vi "Week_4_4.1_Ex-4.vi"() -> ()   [LabVIEW 2015]
panel:
  in  "Gauge":dbl(knob) scale=-360.0..360.0
  out "Active Power":dbl format="%#_13g"
  out "Reactive Power":dbl format="%#_13g"
  out "V RMS":dbl format="%#_13g"
  out "Apparent Power":dbl format="%#_13g"
  out "I-RMS":dbl format="%#_13g"
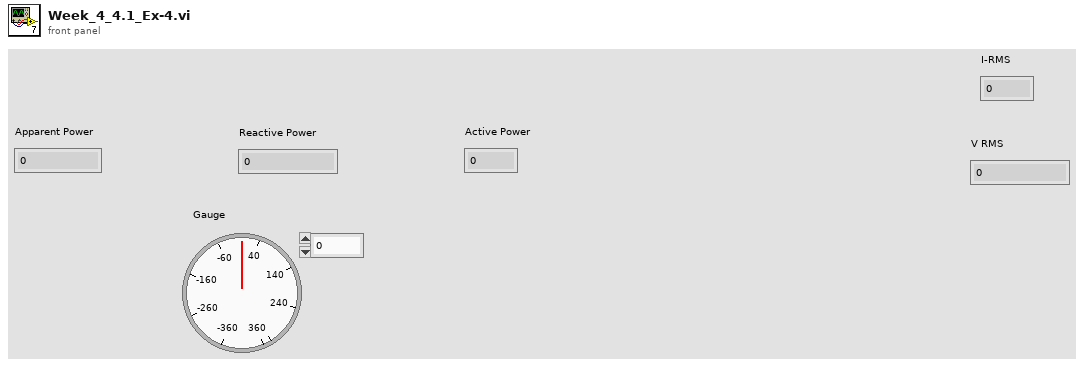
[diagram p1: front panel]
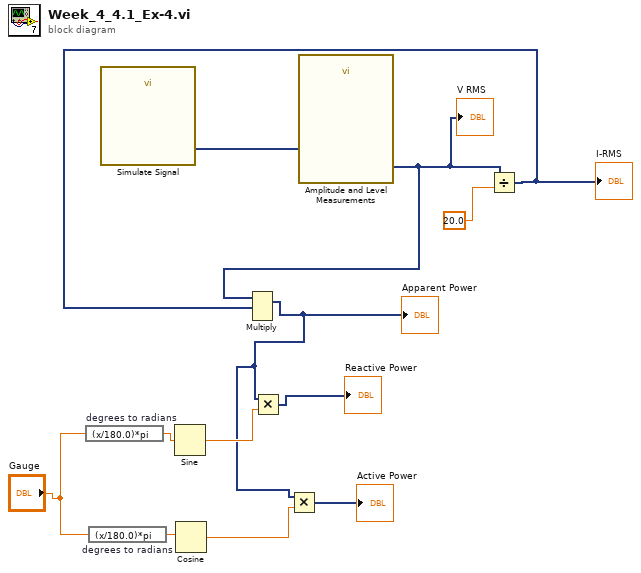
[diagram p0: block diagram]
diagram:
  n1 = expression code="(x/180.0)*pi" "degrees to radians"("Gauge") -> (w3:dbl)
  n2 = expression code="(x/180.0)*pi" "degrees to radians"("Gauge") -> (w4:dbl)
  n3 = call "Simulate Signal"() -> ("Sine"=w11:dynamicdata)  [unwired: 14 in, 1 out]
  n4 = Sine(x=w3) -> (sin(x)=w8:dbl)
  n5 = Cosine(x=w4) -> (cos(x)=w6:dbl)
  n6 = call "Amplitude and Level Measurements"("Signals"=w11) -> ("RMS"=w9:dynamicdata)  [unwired: 13 in, 1 out]
  "V RMS" <- w9
  n7 = Divide(x=w9, y=20.0) -> (x/y=w10:dynamicdata)
  "I-RMS" <- w10
  n8 = Multiply(1:w10, 2:w9) -> (0:w5:dynamicdata)  [unwired: 1 in, 1 out]
  "Apparent Power" <- w5
  n9 = Multiply(x=w5, y=w8) -> (x*y=→"Reactive Power":dynamicdata)
  n10 = Multiply(x=w5, y=w6) -> (x*y=→"Active Power":dynamicdata)
